vi "AlliGator Get-Set State Indicators.vi"(1 "# Defined IRFs":i32, 5 "State Indicators Refnum":refnum<vi>, 7 "AlliGator State Indicators List":T2, 9 "Error In":errorcluster, 12 "ON/OFF":bool, 14 "Set (T)/Get":bool=TRUE) -> (6 "State Indicators Refnum":refnum<vi>, 8 "State Indicator Values":T1 caption="State Indicators", 10 "Error Out":errorcluster)   [LabVIEW 2021, in "AlliGator GUI.lvlib"]
doc: "Gets-sets the requested status LED."
uses:
  AlliGator GUI.lvlib
  AlliGator State Indicator.ctl
  AlliGator State Indicators List.ctl
  5900294e-5d5b-438a-8035-611245816a61.vi
  AlliGator Action Engine.lvlib
panel:
  out "Individual IRFs Defined":bool
  # "see the AlliGator License on the block diagram (Ctrl+E or Window:Show Block Diagram)"
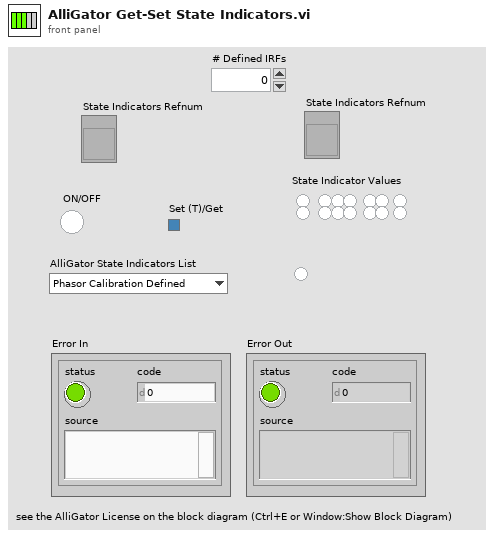
[diagram p1: front panel]
types:
  T1 = typedef "AlliGator GUI.lvlib/AlliGator State Indicator.ctl" = cluster{"Phasor Calibration Defined":bool, "Phasor Calibration Series Defined":bool, "Phasor Calibration Map Defined":bool, "Phasor Ratio Reference 1 Defined":bool, "Phasor Ratio Reference 2 Defined":bool, "Phasor Ratio Lifetime Reference 1 Defined ":bool, "Phasor Ratio Lifetime Reference 2 Defined":bool, "Phasor Calibration Used":bool, "Phasor Calibration Series Used":bool, "Phasor Calibration Map Used":bool, "Dataset Update Needed":bool, "Phasor Plot Update Needed":bool, "Reference/IRF Defined":bool, "Individual IRFs Defined":bool}
  T2 = typedef "AlliGator Action Engine.lvlib/AlliGator State Indicators List.ctl" = enum16{"Phasor Calibration Defined", "Phasor Calibration Series Defined", "Phasor Calibration Map Defined", "Phasor Reference 1 Defined", "Phasor Reference 2 Defined", "Lifetime Reference 1 Defined", "Lifetime Reference 2 Defined", "Phasor Calibration Used", "Phasor Calibration Series Used", "Phasor Calibration Map Used", "Dataset Update Needed", "Phasor Plot Update Needed", "Reference/IRF Defined", "Individual IRFs Defined"}
  T3 = typedef "AlliGator State Indicator.ctl" = cluster{"Phasor Calibration Defined":bool, "Phasor Calibration Series Defined":bool, "Phasor Calibration Map Defined":bool, "Phasor Ratio Reference 1 Defined":bool, "Phasor Ratio Reference 2 Defined":bool, "Phasor Ratio Lifetime Reference 1 Defined ":bool, "Phasor Ratio Lifetime Reference 2 Defined":bool, "Phasor Calibration Used":bool, "Phasor Calibration Series Used":bool, "Phasor Calibration Map Used":bool, "Dataset Update Needed":bool, "Phasor Plot Update Needed":bool, "Reference/IRF Defined":bool, "Individual IRFs Defined":bool}
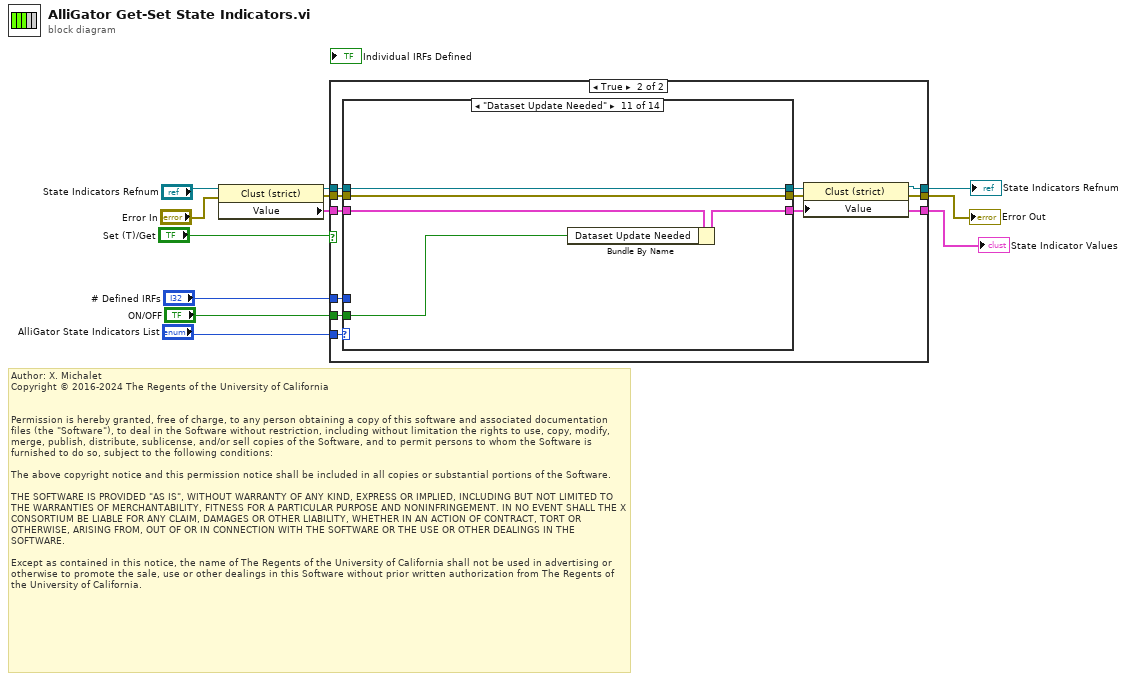
[diagram p0: block diagram]
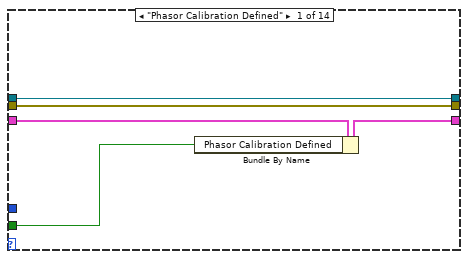
[diagram p3: hidden frame]
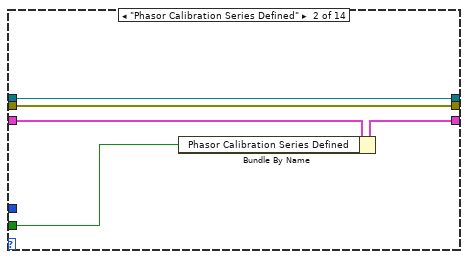
[diagram p4: hidden frame]
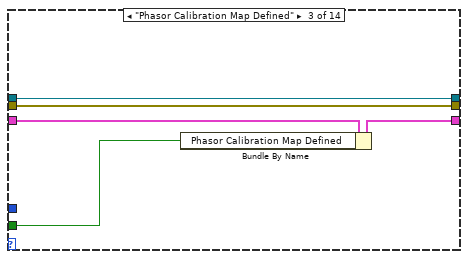
[diagram p5: hidden frame]
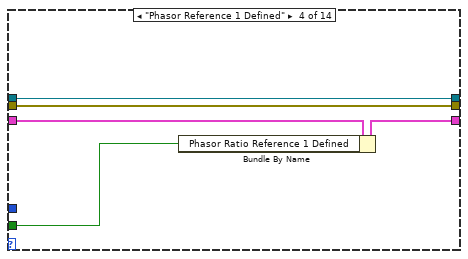
[diagram p6: hidden frame]
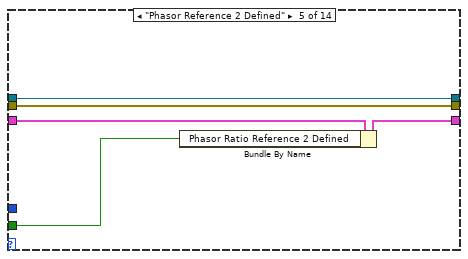
[diagram p7: hidden frame]
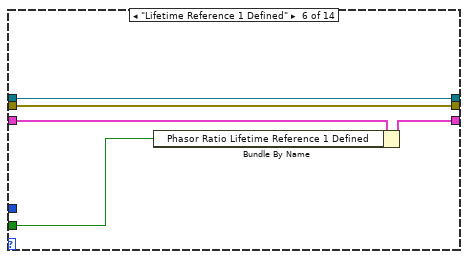
[diagram p8: hidden frame]
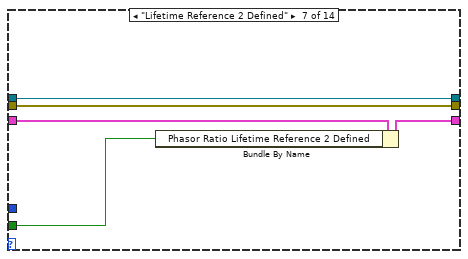
[diagram p9: hidden frame]
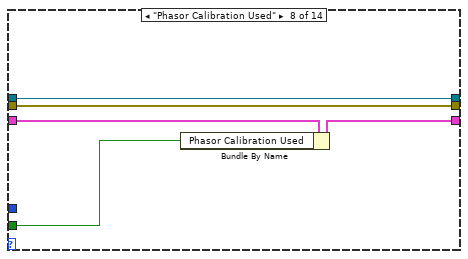
[diagram p10: hidden frame]
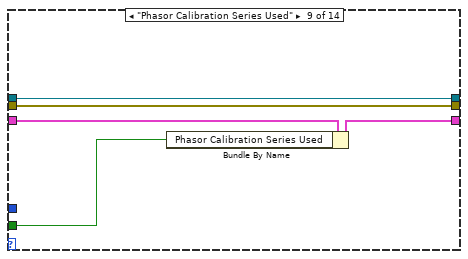
[diagram p11: hidden frame]
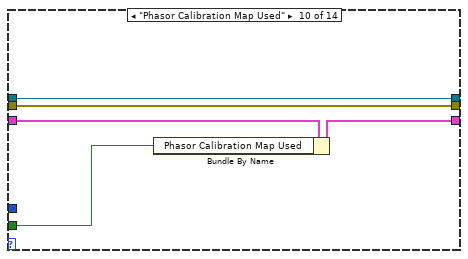
[diagram p12: hidden frame]
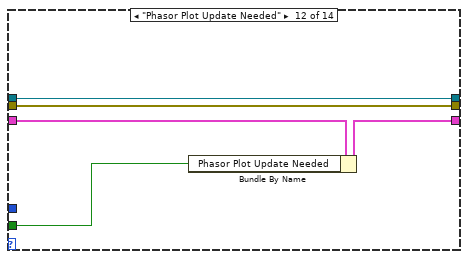
[diagram p13: hidden frame]
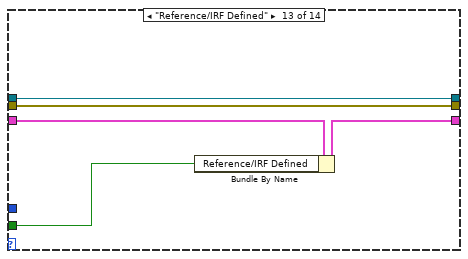
[diagram p14: hidden frame]
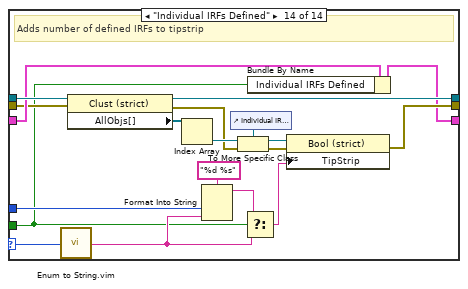
[diagram p15: hidden frame]
diagram:
  # "Author: X. Michalet\nCopyright © 2016-2024 The Regents of the University of California\n \n\nPermission is hereby granted, free of charge, to any person obtaining a copy of this software and associated documentation files (the \"Software\"), to deal in the Software without restriction, including without limitation the rights to use, copy, modify, merge, publish, distribute, sublicense, and/or sell copies of the Software, and to permit persons to whom the Software is furnished to do so, subject to the following conditions:\n\nThe above copyright notice and this permission notice shall be included in all copies or substantial portions of the Software.\n\nTHE SOFTWARE IS PROVIDED \"AS IS\", WITHOUT WARRANTY OF ANY KIND, EXPRESS OR IMPLIED, INCLUDING BUT NOT LIMITED TO THE WARRANTIES OF MERCHANTABILITY, FITNESS FOR A PARTICULAR PURPOSE AND NONINFRINGEMENT. IN NO EVENT SHALL THE X CONSORTIUM BE LIABLE FOR ANY CLAIM, DAMAGES OR OTHER LIABILITY, WHETHER IN AN ACTION OF CONTRACT, TORT OR OTHERWISE, ARISING FROM, OUT OF OR IN CONNECTION WITH THE SOFTWARE OR THE USE OR OTHER DEALINGS IN THE SOFTWARE.\n\nExcept as contained in this notice, the name of The Regents of the University of California shall not be used in advertising or otherwise to promote the sale, use or other dealings in this Software without prior written authorization from The Regents of the University of California."
  n1 = property class="Clust (strict)"(reference="State Indicators Refnum", error in="Error In") -> (reference out=w7:refnum<vi>, error out=w6:errorcluster, "Value"=w11:T3)
  n2 = case shown="True" "Set (T)/Get" {
    tunnel: w11 -> [w15 w26]
    tunnel: "AlliGator State Indicators List" -> [_ w25]
    tunnel: "ON/OFF" -> [_ w24]
    tunnel: w7 -> [w13 w20]
    tunnel: w6 -> [w14 w16]
    tunnel: [w14 w23] -> w5
    tunnel: [w13 w22] -> w4
    tunnel: [w15 w21] -> w3
    tunnel: "# Defined IRFs" -> [_ w17]
    frame False {
    }
    frame True {
      n3 = case shown="\"Dataset Update Needed\"" w25 {
        selector: w25 -> [_ _ _ _ _ _ _ _ _ _ _ _ _ w99]
        tunnel: w26 -> [w31 w36 w41 w46 w51 w56 w61 w66 w71 w76 w81 w86 w91 w108]
        tunnel: w24 -> [w30 w35 w40 w45 w50 w55 w60 w65 w70 w75 w80 w85 w90 w92]
        tunnel: [w29 w34 w39 w44 w49 w54 w59 w64 w69 w74 w79 w84 w89 w100] -> w21
        tunnel: w20 -> [w28 w33 w38 w43 w48 w53 w58 w63 w68 w73 w78 w83 w88 w110]
        tunnel: [w28 w33 w38 w43 w48 w53 w58 w63 w68 w73 w78 w83 w88 w109] -> w19
        tunnel: [w27 w32 w37 w42 w47 w52 w57 w62 w67 w72 w77 w82 w87 w101] -> w18
        tunnel: w17 -> [_ _ _ _ _ _ _ _ _ _ _ _ _ w94]
        tunnel: w16 -> [w27 w32 w37 w42 w47 w52 w57 w62 w67 w72 w77 w82 w87 w93]
        frame "Phasor Calibration Defined" {
          n4 = Bundle By Name(cluster=w31, "Phasor Calibration Defined"=w30) -> (w29:T3)
        }
        frame "Phasor Calibration Series Defined" {
          n5 = Bundle By Name(cluster=w36, "Phasor Calibration Series Defined"=w35) -> (w34:T3)
        }
        frame "Phasor Calibration Map Defined" {
          n6 = Bundle By Name(cluster=w41, "Phasor Calibration Map Defined"=w40) -> (w39:T3)
        }
        frame "Phasor Reference 1 Defined" {
          n7 = Bundle By Name(cluster=w46, "Phasor Ratio Reference 1 Defined"=w45) -> (w44:T3)
        }
        frame "Phasor Reference 2 Defined" {
          n8 = Bundle By Name(cluster=w51, "Phasor Ratio Reference 2 Defined"=w50) -> (w49:T3)
        }
        frame "Lifetime Reference 1 Defined" {
          n9 = Bundle By Name(cluster=w56, "Phasor Ratio Lifetime Reference 1 Defined"=w55) -> (w54:T3)
        }
        frame "Lifetime Reference 2 Defined" {
          n10 = Bundle By Name(cluster=w61, "Phasor Ratio Lifetime Reference 2 Defined"=w60) -> (w59:T3)
        }
        frame "Phasor Calibration Used" {
          n11 = Bundle By Name(cluster=w66, "Phasor Calibration Used"=w65) -> (w64:T3)
        }
        frame "Phasor Calibration Series Used" {
          n12 = Bundle By Name(cluster=w71, "Phasor Calibration Series Used"=w70) -> (w69:T3)
        }
        frame "Phasor Calibration Map Used" {
          n13 = Bundle By Name(cluster=w76, "Phasor Calibration Map Used"=w75) -> (w74:T3)
        }
        frame "Dataset Update Needed" {
          n14 = Bundle By Name(cluster=w81, "Dataset Update Needed"=w80) -> (w79:T3)
        }
        frame "Phasor Plot Update Needed" {
          n15 = Bundle By Name(cluster=w86, "Phasor Plot Update Needed"=w85) -> (w84:T3)
        }
        frame "Reference/IRF Defined" {
          n16 = Bundle By Name(cluster=w91, "Reference/IRF Defined"=w90) -> (w89:T3)
        }
        frame "Individual IRFs Defined" {
          # "Adds number of defined IRFs to tipstrip"
          n17 = call "Enum to String.vim"("Enum"=w99) -> ("String"=w97:string)
          n18 = property class="Clust (strict)"(reference=w110, error in=w93) -> (reference out=w109:refnum<vi>, error out=w103:errorcluster, "AllObjs[]"=w107:refnum<vi>[])
          n19 = Index Array(array=w107) -> (element=w106:refnum<vi>)  [unwired: 1 in]
          n20 = Format Into String(format string="%d %s", w94, w97) -> (resulting string=w96:string)  [unwired: 2 in, 1 out]
          n21 = control-ref of="Individual IRFs Defined"() -> (w104:refnum<vi>)
          n22 = To More Specific Class(target class=w104, reference=w106, error in=w103) -> (specific class reference=w105:refnum<vi>, error out=w102:errorcluster)
          n23 = Select(t=w96, s=w92, f=w97) -> (s? t:f=w98:string)
          n24 = Bundle By Name(cluster=w108, "Individual IRFs Defined"=w92) -> (w100:T3)
          n25 = property class="Bool (strict)"(reference=w105, error in=w102, "TipStrip"=w98) -> (error out=w101:errorcluster)  [unwired: 1 out]
        }
      }
      n26 = property class="Clust (strict)"(reference=w19, error in=w18, "Value"=w21) -> (reference out=w22:refnum<vi>, error out=w23:errorcluster)
    }
  }
  "Error Out" <- w5
  "State Indicators Refnum" <- w4
  "State Indicator Values" <- w3
